vi "currentVariant.vi"() -> ()   [LabVIEW 2018]
uses:
  <vilib>/Analysis/baseanly.llb/Mean (DBL).vi
  Projects/1259_usbComm/#include/Global_usbComm.vi
  <vilib>/Analysis/NI_AALBase.lvlib
panel:
  out "BaseCurrent":string
  out "currentMaxFan":string
  in  "FAN1":bool
  in  "FAN0":bool
  out "FanCurrent":dbl(graph)
  out "Ifan":string
  out "limitFan":bool
  out "FAN-18":string
  out "fanIPeak":string
  in  "EQF1259 com port":refnum<visa-resource-name>
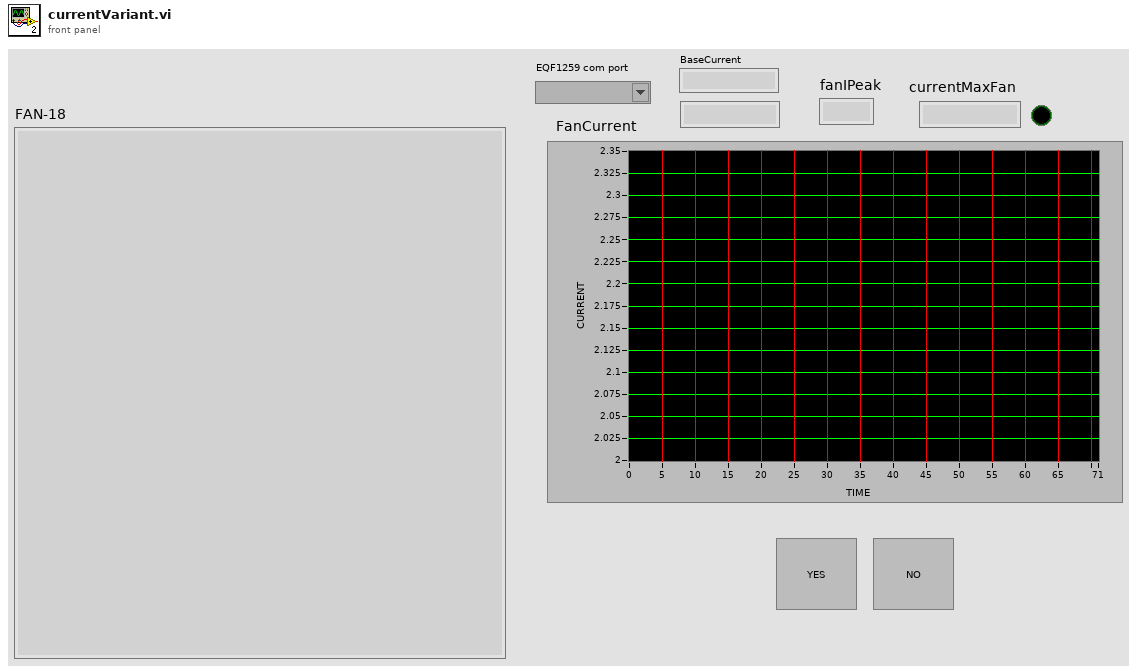
[diagram p1: front panel]
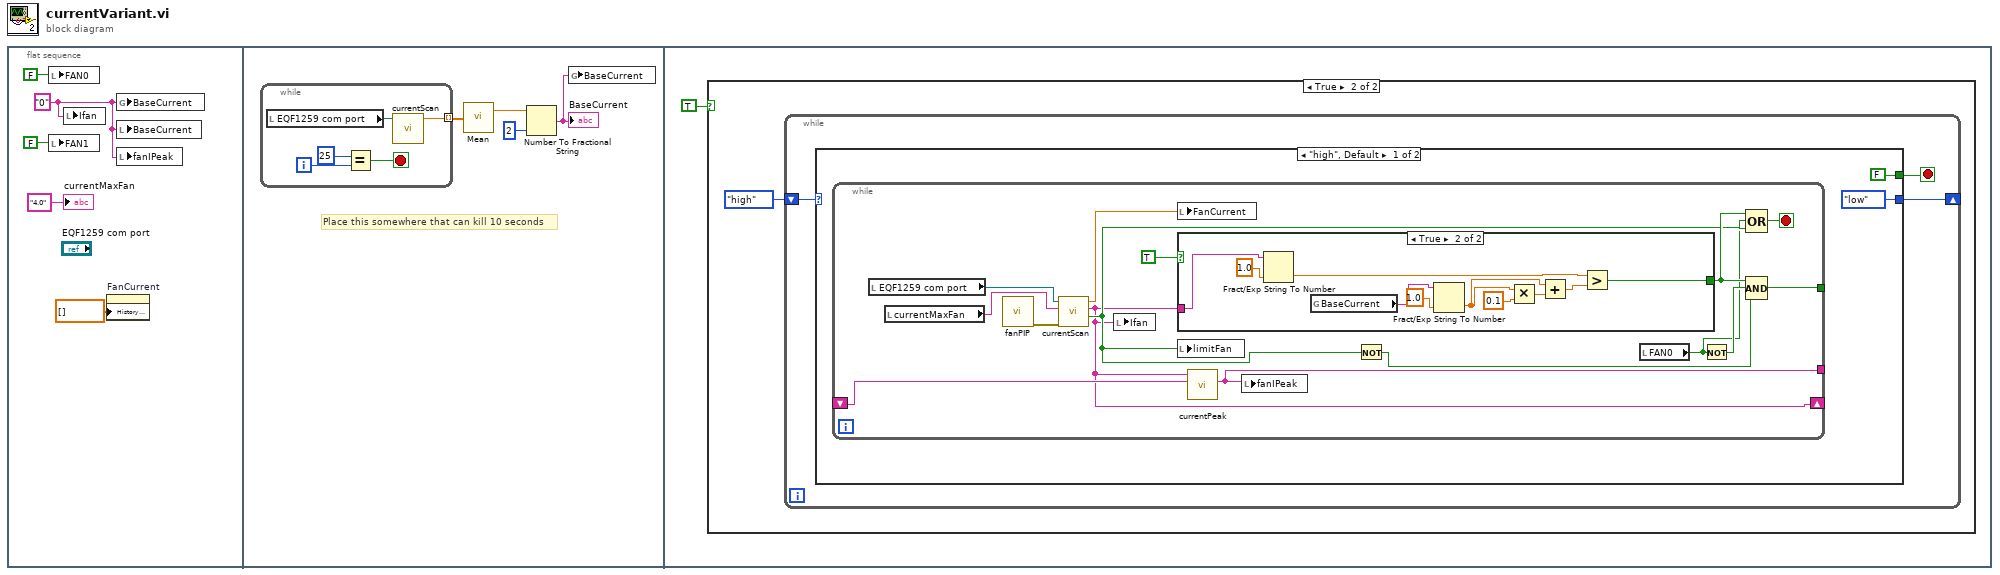
[diagram p0: block diagram]
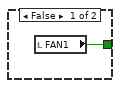
[diagram p3: hidden frame]
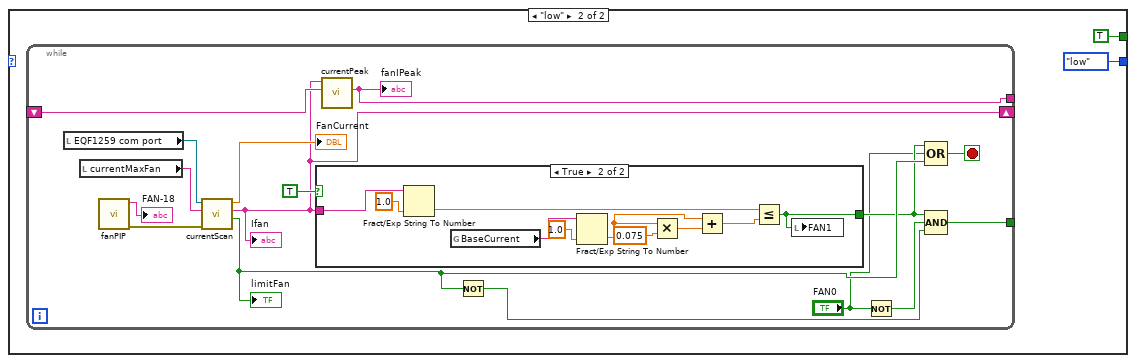
[diagram p4: hidden frame]
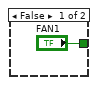
[diagram p5: hidden frame]
diagram:
  n1 = flat-sequence {
    frame #0 {
      w2 = "0" ("fanIPeak")
      n2 = local write "FAN0"(FALSE ("FAN0")) -> ()
      n3 = local write "FAN1"(FALSE ("FAN0")) -> ()
      n4 = local write "Ifan"(w2) -> ()
      n5 = property on="FanCurrent" class="WFChart (strict)"("History Data"=dbl[] []) -> ()  [unwired: 2 in, 2 out]
      n6 = global write "Global_usbComm.vi" "BaseCurrent"(w2) -> ()
      n7 = local write "BaseCurrent"(w2) -> ()
      n8 = local write "fanIPeak"(w2) -> ()
      "currentMaxFan" <- "4.0" ("currentMaxFan")
    }
    frame #1 {
      # "Place this somewhere that can kill 10 seconds"
      n9 = while {
        tunnel: [w13] -> w7 mode=indexing
        i -> [w11]
        stop <- w12 stop-if-true
        n10 = local read "EQF1259 com port"() -> (w14:refnum<visa-resource-name>)
        n11 = Equal?(x=25, y=w11) -> (x = y?=w12:bool)
        n12 = call "currentScan.vi"("VISA resource name"=w14) -> ("Ichart"=w13:dbl)  [unwired: 7 in, 3 out]
      }
      n13 = call-poly <vilib>:"Mean.vi"("X"=w7) -> ("mean"=w8:dbl)  [unwired: 1 out]
      n14 = Number To Fractional String(number=w8, precision (6)=i16 2) -> (F-format string=w9:string)  [unwired: 2 in]
      "BaseCurrent" <- w9
      n15 = global write "Global_usbComm.vi" "BaseCurrent"(w9) -> ()
    }
    frame #2 {
      n16 = case shown="True" TRUE {
        frame False {
        }
        frame True {
          n17 = while {
            shift-right: [w18] -> _
            shift-left: enum16{"high", "low"}."high" -> [w19]
            stop <- w17 stop-if-true
            n18 = case shown="\"high\", Default" w19 {
              tunnel: [enum16{"high", "low"}."low" enum16{"high", "low"}."low"] -> w18
              tunnel: [FALSE TRUE] -> w17
              frame "high", Default {
                n19 = while {
                  tunnel: [w32] -> _
                  shift-right: [w24] -> _
                  shift-left: _ -> [w29]
                  tunnel: [w26] -> _
                  stop <- w36 stop-if-true
                  n20 = local read "EQF1259 com port"() -> (w35:refnum<visa-resource-name>)
                  n21 = local read "currentMaxFan"() -> (w34:string)
                  n22 = call "fanPIP.vi"() -> ("error out"=w33:errorcluster)  [unwired: 10 in, 1 out]
                  n23 = call "currentScan.vi"("error in (no error)"=w33, "Imax"=w34, "VISA resource name"=w35) -> ("max"=w25:bool, "Istring"=w24:string, "Ichart"=w23:dbl)  [unwired: 5 in, 1 out]
                  n24 = local write "Ifan"(w24) -> ()
                  n25 = local write "FanCurrent"(w23) -> ()
                  n26 = case shown="True" TRUE {
                    tunnel: [w37 w38] -> w27
                    tunnel: w24 -> [_ w41]
                    frame False {
                      n27 = local read "FAN1"() -> (w37:bool)
                    }
                    frame True {
                      n28 = Fract/Exp String To Number(string=w41, default (0 dbl)=1.0 ("default (0 DBL)")) -> (number=w40:dbl)  [unwired: 2 in, 1 out]
                      n29 = global read "Global_usbComm.vi" "BaseCurrent"() -> (w47:string)
                      n30 = Fract/Exp String To Number(string=w47, default (0 dbl)=1.0 ("default (0 DBL)")) -> (number=w43:dbl)  [unwired: 2 in, 1 out]
                      n31 = Multiply(x=w43, y=0.1) -> (x*y=w44:dbl)
                      n32 = Add(x=w43, y=w44) -> (x+y=w42:dbl)
                      n33 = Greater?(x=w40, y=w42) -> (0:w38:bool)
                    }
                  }
                  n34 = local write "limitFan"(w25) -> ()
                  n35 = call "currentPeak.vi"("Istring# change"=w29, "Istring# scan"=w24) -> ("Ipeak"=w26:string)  [unwired: 7 in, 2 out]
                  n36 = local write "fanIPeak"(w26) -> ()
                  n37 = Not(x=w25) -> (.not. x?=w30:bool)
                  n38 = local read "FAN0"() -> (w22:bool)
                  n39 = Not(x=w22) -> (.not. x?=w31:bool)
                  n40 = Compound Arithmetic op=OR(w27, w22, w25) -> (w36:bool)
                  n41 = Compound Arithmetic op=AND(w27, w31, w30) -> (w32:bool)
                }
              }
              frame "low" {
                n42 = while {
                  tunnel: [w59] -> _
                  shift-right: [w51] -> _
                  shift-left: _ -> [w56]
                  tunnel: [w55] -> _
                  stop <- w65 stop-if-true
                  n43 = local read "EQF1259 com port"() -> (w64:refnum<visa-resource-name>)
                  n44 = local read "currentMaxFan"() -> (w63:string)
                  n45 = call "fanPIP.vi"() -> ("error out"=w61:errorcluster, "FAN-18"=→"FAN-18":string)  [unwired: 10 in]
                  n46 = call "currentScan.vi"("error in (no error)"=w61, "Imax"=w63, "VISA resource name"=w64) -> ("max"=w62:bool, "Istring"=w51:string, "Ichart"=→"FanCurrent":dbl)  [unwired: 5 in, 1 out]
                  "Ifan" <- w51
                  "limitFan" <- w62
                  n47 = case shown="True" TRUE {
                    tunnel: ["FAN1" w67] -> w52
                    tunnel: w51 -> [_ w70]
                    frame False {
                    }
                    frame True {
                      n48 = Fract/Exp String To Number(string=w70, default (0 dbl)=1.0 ("default (0 DBL)")) -> (number=w69:dbl)  [unwired: 2 in, 1 out]
                      n49 = global read "Global_usbComm.vi" "BaseCurrent"() -> (w76:string)
                      n50 = Fract/Exp String To Number(string=w76, default (0 dbl)=1.0 ("default (0 DBL)")) -> (number=w72:dbl)  [unwired: 2 in, 1 out]
                      n51 = Multiply(x=w72, y=0.075) -> (x*y=w73:dbl)
                      n52 = Add(x=w72, y=w73) -> (x+y=w71:dbl)
                      n53 = Less Or Equal?(x=w69, y=w71) -> (x <= y?=w67:bool)
                      n54 = local write "FAN1"(w67) -> ()
                    }
                  }
                  n55 = call "currentPeak.vi"("Istring# change"=w56, "Istring# scan"=w51) -> ("Ipeak"=w55:string)  [unwired: 7 in, 2 out]
                  "fanIPeak" <- w55
                  n56 = Not(x=w62) -> (.not. x?=w57:bool)
                  n57 = Not(x="FAN0") -> (.not. x?=w58:bool)
                  n58 = Compound Arithmetic op=OR(w52, "FAN0", w62) -> (w65:bool)
                  n59 = Compound Arithmetic op=AND(w52, w58, w57) -> (w59:bool)
                }
              }
            }
          }
        }
      }
    }
  }
